vi "getDevice.vi"(8 "error in (no error)":errorcluster, 11 "DeviceData.lvclass in":refnum<class "DeviceData.lvclass">) -> (0 "error out":errorcluster, 2 "device":refnum<class "device.lvclass">, 3 "DeviceData.lvclass out":refnum<class "DeviceData.lvclass">)   [LabVIEW 2009, in "DataMappers.lvlib" / "DeviceData.lvclass"]
uses:
  DeviceData.lvclass
  DatabaseHelpers/Database Objects/device/device.lvclass
  DeviceData.lvclass/DeviceData.ctl
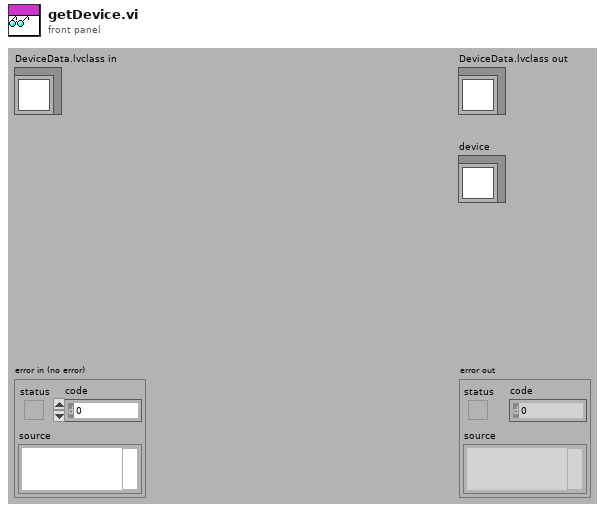
[diagram p1: front panel]
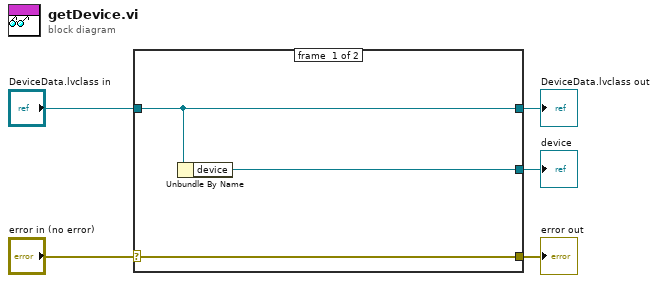
[diagram p0: block diagram]
diagram:
  n1 = case shown="No Error" "error in (no error)" {
    selector: "error in (no error)" -> [w8 w9]
    tunnel: [w8 w9] -> w4
    tunnel: [w7 w10] -> w2
    tunnel: "DeviceData.lvclass in" -> [w7 w10]
    tunnel: [w6 _] -> w1
    frame #0 {
      n2 = Unbundle By Name(w7) -> ("device"=w6:refnum<class "device.lvclass">)
    }
    frame #1 {
    }
  }
  "error out" <- w4
  "DeviceData.lvclass out" <- w2
  "device" <- w1
